vi "DSF.Engine.Pointer.DBL.New.vi"(8 "error in (no error)":errorcluster, 11 "channel count":u64) -> (0 "error out":errorcluster, 3 "DBL Pointer out":refnum<class "DSF.Engine.Pointer.DBL.lvclass">)   [LabVIEW 2017, in "DSF.Engine.lvlib" / "DSF.Engine.Pointer.DBL.lvclass"]
uses:
  DSF.Engine.Pointer.DBL.lvclass
  C:/Program Files (x86)/National Instruments/LabVIEW 2017/vi.lib/National Instruments/Memory Manager/Classes/Pointer/Memory.Pointer.lvclass
  DSF.Engine.Pointer.DBL.lvclass/DSF.Engine.Pointer.DBL.ctl
  <vilib>/National Instruments/Memory Manager/Classes/Pointer/Memory.Pointer.lvclass/Memory.Pointer.ctl
  <vilib>/National Instruments/Memory Manager/Classes/Pointer/Memory.Pointer.New.8B.vi
  <vilib>/National Instruments/Memory Manager/Classes/Pointer/Memory.Pointer.Allocate.vi
  <vilib>/National Instruments/Memory Manager/Classes/Pointer/Memory.Pointer.Set Address.vi
  <vilib>/National Instruments/Memory Manager/Classes/Pointer/Memory.Pointer.Set Size.vi
  <vilib>/National Instruments/Memory Manager/Classes/Pointer/Memory.Pointer.Set Allocated.vi
  <vilib>/National Instruments/Memory Manager/Classes/Pointer/Memory.Pointer.lvclass
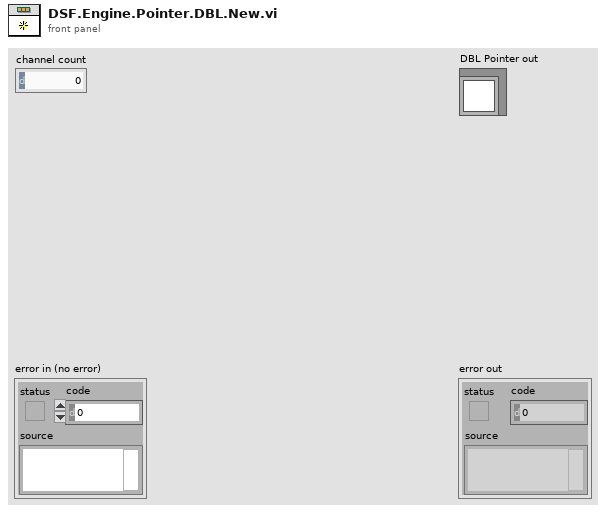
[diagram p1: front panel]
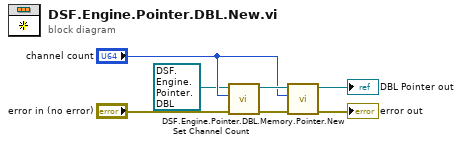
[diagram p0: block diagram]
diagram:
  n1 = call "DSF.Engine.Pointer.DBL.Set Channel Count.vi"("channel count"="channel count", "DBL Buffer in"=refnum<class "DSF.Engine.Pointer.DBL.lvclass"> refnum) -> ("DBL Buffer out"=w6:refnum<class "DSF.Engine.Pointer.DBL.lvclass">)  [unwired: 9 in]
  n2 = call-poly <vilib>:"Memory.Pointer.New.vi"("error in (no error)"="error in (no error)", "count (1)"="channel count", "Pointer type"=w6) -> ("error out"=→"error out":errorcluster, "Pointer"=→"DBL Pointer out":refnum<class "DSF.Engine.Pointer.DBL.lvclass">)  [unwired: 7 in]
